vi "dfd_Validate Moving Average FXP for Code Gen.vi"(7 "totalChan":i32=3, 8 "error in":errorcluster, 11 "multirate filter":T1={"mMRate_Structure"=enum."CIC", "mMRate_Mode"=0, "mMRate_Factor"=1, "mMRate_FIRParams"={"mMRate_FIR_H"=[], "mMRate_FIR_IsNyquist?"=FALSE, "mMRate_FIR_IsSymmetric?"=FALSE}, "mMRate_CICParams"={"mMRate_CIC_#Stage"=2, "mMRate_CIC_Lag"=1, "mMRate_CIC_Type"=enum."Lowpass"}, "mMRate_Order"=0, "mMRate_Version"="1.0", "mMRate_Comments"="", "mMRate_RationalFactor"={"mMRate_L"=-1, "mMRate_M"=-1}, "mMRate_Fs"=1.0, "mMRate_Quantized?"=FALSE, "mMRate_QFilterGain"=1.0, "mMRate_CoefWl"=16, "mMRate_Scaling"={"mMRate_ScaleByPowerOf2?"=FALSE, "mMRate_ScaleType"=enum."Time Domain 1-Norm"}, "mMRate_InputWl"=0, "mMRate_OutputWl"=0, "mMRate_OutputMode"=enum."Nearest", "mMRate_MultMode"=enum."Truncated", "mMRate_BitPruning"=FALSE, "mMRate_GainWl"=16, "mMRate_OutputFwl"=0, "mMRate_SumIwl"=0, "mMRate_InputIwl "=16, "mMRate_SumWl"=32, "mMRate_CoefIwl"=0} {"mMRate_SumWl" min=1 max=32 step=1; "mMRate_InputIwl" min=1 max=32 step=1; "mMRate_GainWl" min=1 max=32 step=1; "mMRate_OutputWl" min=1 max=32 step=1; "mMRate_InputWl" min=1 max=32 step=1; "mMRate_CoefWl" min=1 max=32 step=1; "mMRate_Mode" items=["Default"=-1, "No Rate Change"=0, "Interpolation"=1, "Decimation"=2, "Interpolated"=3, "Rational"=4]}) -> (0 "error out":errorcluster, 3 "multirate filter out":T1={"mMRate_Structure"=enum."CIC", "mMRate_Mode"=0, "mMRate_Factor"=1, "mMRate_FIRParams"={"mMRate_FIR_H"=[], "mMRate_FIR_IsNyquist?"=FALSE, "mMRate_FIR_IsSymmetric?"=FALSE}, "mMRate_CICParams"={"mMRate_CIC_#Stage"=2, "mMRate_CIC_Lag"=1, "mMRate_CIC_Type"=enum."Lowpass"}, "mMRate_Order"=0, "mMRate_Version"="1.0", "mMRate_Comments"="", "mMRate_RationalFactor"={"mMRate_L"=-1, "mMRate_M"=-1}, "mMRate_Fs"=1.0, "mMRate_Quantized?"=FALSE, "mMRate_QFilterGain"=1.0, "mMRate_CoefWl"=16, "mMRate_Scaling"={"mMRate_ScaleByPowerOf2?"=FALSE, "mMRate_ScaleType"=enum."Time Domain 1-Norm"}, "mMRate_InputWl"=0, "mMRate_OutputWl"=0, "mMRate_OutputMode"=enum."Nearest", "mMRate_MultMode"=enum."Truncated", "mMRate_BitPruning"=FALSE, "mMRate_GainWl"=16, "mMRate_OutputFwl"=0, "mMRate_SumIwl"=0, "mMRate_InputIwl "=16, "mMRate_SumWl"=32, "mMRate_CoefIwl"=0} {"mMRate_SumWl" min=1 max=32 step=1; "mMRate_InputIwl" min=1 max=32 step=1; "mMRate_GainWl" min=1 max=32 step=1; "mMRate_OutputWl" min=1 max=32 step=1; "mMRate_InputWl" min=1 max=32 step=1; "mMRate_CoefWl" min=1 max=32 step=1; "mMRate_Mode" items=["Default"=-1, "No Rate Change"=0, "Interpolation"=1, "Decimation"=2, "Interpolated"=3, "Rational"=4]})   [LabVIEW 2017, in "NI_DigFilterLicensed.lvlib"]
uses:
  <vilib>/addons/Digital Filter Design/NI_DigFilterLicensed.lvlib
  <vilib>/addons/Digital Filter Design/_Objects.llb/DFD Multirate Filter Obj.ctl
  <vilib>/addons/Digital Filter Design/_Objects.llb/DFD Multirate Mode.ctl
  <vilib>/addons/Digital Filter Design/_Objects.llb/DFD Coef Norm Type.ctl
  <vilib>/addons/Digital Filter Design/_Objects.llb/DFD Round-off Mode.ctl
  <vilib>/addons/Digital Filter Design/_Objects.llb/DFD FXP MRate Multiply Mode.ctl
  <vilib>/addons/Digital Filter Design/_Misc.llb/dfd_Error Handlers (Single).vi
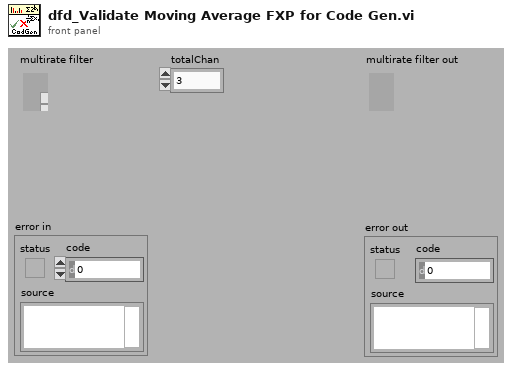
[diagram p1: front panel]
types:
  T1 = typedef "NI_DigFilterLicensed.lvlib/DFD Multirate Filter Obj.ctl" = cluster{"mMRate_Structure":enum16{"CIC", "FIR", "IIR", "Lattice"}, "mMRate_Mode":T2, "mMRate_Factor":i32, "mMRate_FIRParams":cluster{"mMRate_FIR_H":dbl[], "mMRate_FIR_IsNyquist?":bool, "mMRate_FIR_IsSymmetric?":bool}, "mMRate_CICParams":cluster{"mMRate_CIC_#Stage":i32, "mMRate_CIC_Lag":i32, "mMRate_CIC_Type":enum16{"Lowpass", "Highpass"}}, "mMRate_Order":i32, "mMRate_Version":string, "mMRate_Comments":string, "mMRate_RationalFactor":cluster{"mMRate_L":i32, "mMRate_M":i32}, "mMRate_Fs":dbl, "mMRate_Quantized?":bool, "mMRate_QFilterGain":dbl, "mMRate_CoefWl":i16, "mMRate_Scaling":cluster{"mMRate_ScaleByPowerOf2?":bool, "mMRate_ScaleType":T3}, "mMRate_InputWl":i16, "mMRate_OutputWl":i16, "mMRate_OutputMode":T4, "mMRate_MultMode":T5, "mMRate_BitPruning":bool, "mMRate_GainWl":i16, "mMRate_OutputFwl":i16, "mMRate_SumIwl":i16, "mMRate_InputIwl ":i16, "mMRate_SumWl":i16, "mMRate_CoefIwl":i16}
  T2 = typedef "NI_DigFilterLicensed.lvlib/DFD Multirate Mode.ctl" = i16
  T3 = typedef "NI_DigFilterLicensed.lvlib/DFD Coef Norm Type.ctl" = enum16{"No Norm", "Time Domain 1-Norm", "Time Domain 2-Norm", "Time Domain Inf-Norm"}
  T4 = typedef "NI_DigFilterLicensed.lvlib/DFD Round-off Mode.ctl" = enum16{"Nearest", "Truncation"}
  T5 = typedef "NI_DigFilterLicensed.lvlib/DFD FXP MRate Multiply Mode.ctl" = enum16{"Truncated", "Full"}
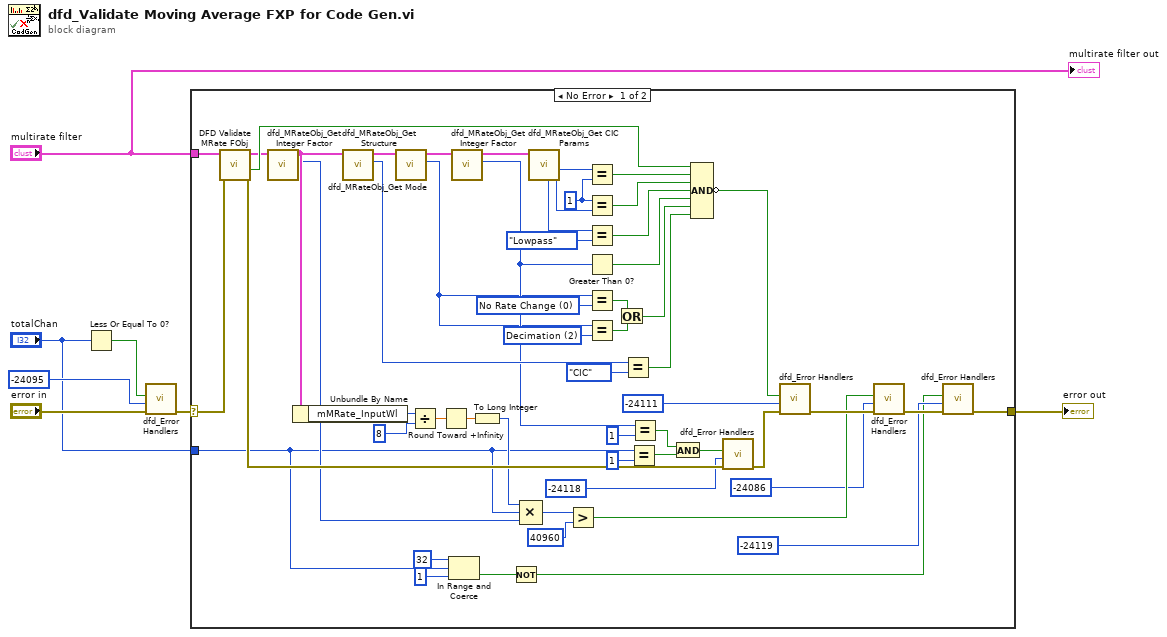
[diagram p0: block diagram]
diagram:
  n1 = Less Or Equal To 0?(x="totalChan") -> (x <= 0?=w2:bool)
  n2 = call-poly <vilib>:"dfd_Error Handlers.vi"("error in (no error)"="error in", "error code"=-24095 ("ERR_SRATE_#CH"), "condition failed?"=w2) -> ("error out"=w4:errorcluster)  [unwired: 8 out]
  n3 = case shown="No Error" w4 {
    selector: w4 -> [w40 w64]
    tunnel: "multirate filter" -> [w29 _]
    tunnel: [w14 w64] -> w7
    tunnel: "totalChan" -> [w12 _]
    frame No Error {
      w57 = T2 2 items=["Default"=-1, "No Rate Change"=0, "Interpolation"=1, "Decimation"=2, "Interpolated"=3, "Rational"=4] ("y")
      w58 = T2 0 items=["Default"=-1, "No Rate Change"=0, "Interpolation"=1, "Decimation"=2, "Interpolated"=3, "Rational"=4] ("y")
      w50 = 1 ("x")
      n4 = call <vilib>:"DFD Validate MRate FObj.vi"("error in (no error)"=w40, "multirate filter in"=w29) -> ("error out"=w33:errorcluster, "is valid FXP?"=w41:bool, "multirate filter out"=w28:T1)  [unwired: 7 out]
      n5 = call <vilib>:"dfd_MRateObj_Get Integer Factor.vi"("multirate filter in"=w28) -> ("factor"=w22:i32, "dup multirate filter"=w27:T1)  [unwired: 9 out]
      n6 = Unbundle By Name(w27) -> ("mMRate_InputWl"=w26:i16)
      n7 = call <vilib>:"dfd_MRateObj_Get Structure.vi"("multirate filter in"=w27) -> ("structure"=w60:enum16{"CIC", "FIR", "IIR", "Lattice"}, "dup multirate filter"=w63:T1)  [unwired: 9 out]
      n8 = call <vilib>:"dfd_MRateObj_Get Mode.vi"("multirate filter in"=w63) -> ("mode"=w30:T2, "dup multirate filter"=w62:T1)  [unwired: 9 out]
      n9 = Divide(x=w26, y=i16 8) -> (x/y=w24:dbl)
      n10 = Round Toward +Infinity(x=w24) -> (ceil(x): smallest int >= x=w23:dbl)
      n11 = In Range and Coerce(upper limit=32 ("totalChan"), x=w12, lower limit=1) -> (In Range?=w9:bool)  [unwired: 1 out]
      n12 = call <vilib>:"dfd_MRateObj_Get Integer Factor.vi"("multirate filter in"=w62) -> ("factor"=w37:i32, "dup multirate filter"=w61:T1)  [unwired: 9 out]
      n13 = To Long Integer(number=w23) -> (32bit integer=w21:i32)
      n14 = Not(x=w9) -> (.not. x?=w8:bool)
      n15 = Compound Arithmetic op=MULTIPLY(w21, w12, w22) -> (w20:i32)
      n16 = call <vilib>:"dfd_MRateObj_Get CIC Params.vi"("multirate filter in"=w61) -> ("lag"=w52:i32, "# stages"=w51:i32, "type"=w54:enum16{"Lowpass", "Highpass"})  [unwired: 8 out]
      n17 = Greater?(x=w20, y=40960) -> (0:w17:bool)
      n18 = Equal?(x=w51, y=w50) -> (x = y?=w49:bool)
      n19 = Equal?(x=w50, y=w52) -> (x = y?=w48:bool)
      n20 = Equal?(x=w54, y=enum16{"Lowpass", "Highpass"}."Lowpass") -> (x = y?=w47:bool)
      n21 = Greater Than 0?(x=w37) -> (x > 0?=w46:bool)
      n22 = Equal?(x=w30, y=w58) -> (x = y?=w56:bool)
      n23 = Equal?(x=w30, y=w57) -> (x = y?=w55:bool)
      n24 = Or(x=w56, y=w55) -> (x .or. y?=w45:bool)
      n25 = Equal?(x=w60, y=enum16{"CIC", "FIR", "IIR", "Lattice"}."CIC") -> (x = y?=w44:bool)
      n26 = Equal?(x=w12, y=1) -> (x = y?=w36:bool)
      n27 = Equal?(x=w37, y=1) -> (x = y?=w35:bool)
      n28 = And(x=w35, y=w36) -> (x .and. y?=w34:bool)
      n29 = Compound Arithmetic op=AND(w41, w49, w48, w47, w46, w45, w44) -> (invert w42:bool)
      n30 = call-poly <vilib>:"dfd_Error Handlers.vi"("error in (no error)"=w33, "error code"=-24118 ("ERR_MA_FACTOR_INVALID"), "condition failed?"=w34) -> ("error out"=w32:errorcluster)  [unwired: 8 out]
      n31 = call-poly <vilib>:"dfd_Error Handlers.vi"("error in (no error)"=w32, "error code"=-24111 ("ERR_NOT_MA"), "condition failed?"=w42) -> ("error out"=w18:errorcluster)  [unwired: 8 out]
      n32 = call-poly <vilib>:"dfd_Error Handlers.vi"("error in (no error)"=w18, "error code"=-24086 ("ERR_MEM_FULL"), "condition failed?"=w17) -> ("error out"=w15:errorcluster)  [unwired: 8 out]
      n33 = call-poly <vilib>:"dfd_Error Handlers.vi"("error in (no error)"=w15, "error code"=-24119 ("ERR_MA_#CH"), "condition failed?"=w8) -> ("error out"=w14:errorcluster)  [unwired: 8 out]
    }
    frame Error {
    }
  }
  "error out" <- w7
  "multirate filter out" <- "multirate filter"
